vi "get sync out settings.vi"(8 "error in (no error)":errorcluster, 10 "sync_out_settings":T1, 11 "id":i32) -> (0 "error out":errorcluster, 2 "sync_out_settings out":T1, 3 "function return":i32)   [LabVIEW 2012, in "libximc.lvlib"]
doc: "result_t XIMC_API get_sync_out_settings (device_t id, sync_out_settings_t* sync_out_settings);"
uses:
  libximc.lvlib
  libximc.dll
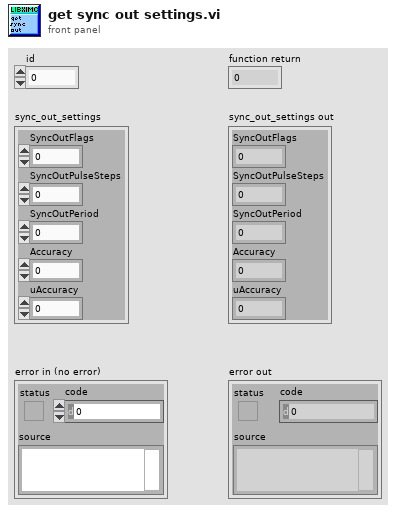
[diagram p1: front panel]
types:
  T1 = cluster{"SyncOutFlags":u32, "SyncOutPulseSteps":u32, "SyncOutPeriod":u32, "Accuracy":u32, "uAccuracy":u32}
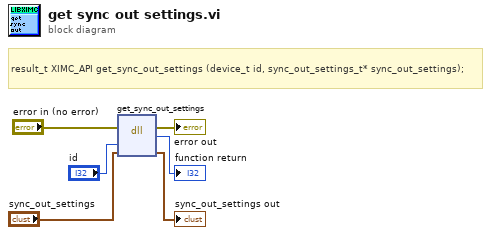
[diagram p0: block diagram]
diagram:
  # "result_t XIMC_API get_sync_out_settings (device_t id, sync_out_settings_t* sync_out_settings);"
  n1 = dll-call lib="E:/labview-2.12.1-Labview_12.0/ximcLVx32/libximc.*" fn="get_sync_out_settings"(error in="error in (no error)", "id"="id", "sync_out_settings"="sync_out_settings") -> (error out=→"error out":errorcluster, →"function return":i32, "sync_out_settings"=→"sync_out_settings out":T1)  [unwired: 3 in, 1 out]
